vi "Configure Regions.vi"(8 "error in (no error)":errorcluster, 10 "regions":T1(array[cluster]), 11 "SOL Camera in":refnum<class "PL SOL Instruments Camera.lvclass">) -> (0 "error out":errorcluster, 3 "SOL Camera out":refnum<class "PL SOL Instruments Camera.lvclass">)   [LabVIEW 2015, in "PL SOL Instruments Camera.lvclass"]
doc: "Configures acquisition regions."
uses:
  PL SOL Instruments Camera.lvclass
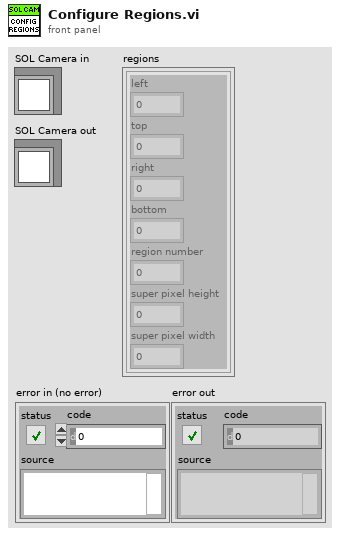
[diagram p1: front panel]
types:
  T1 = cluster{"left":u16, "top":u16, "right":u16, "bottom":u16, "region number":u16, "super pixel height":u16, "super pixel width":u16}[]
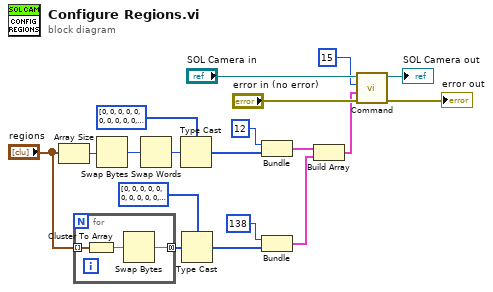
[diagram p0: block diagram]
diagram:
  n1 = Array Size(array="regions") -> (size(s)=w10:i32)
  n2 = for {
    tunnel: "regions" -> [w22] mode=indexing
    tunnel: [w20] -> w5 mode=concatenating
    n3 = Cluster To Array(cluster=w22) -> (array=w21:u16[])
    n4 = Swap Bytes(anything=w21) -> (byte swapped=w20:u16[])
  }
  n5 = Swap Bytes(anything=w10) -> (byte swapped=w12:i32)
  n6 = Swap Words(1:w12) -> (0:w11:i32)
  n7 = Type Cast(type=u8[] [0, 0, 0, 0, 0, 0, 0, 0, 0, 0, 0, 0, 0, 0, 0, 0, 0, 0, 0, 0, 0, 0, 0, 0, 0, 0, 0, 0, 0, 0, 0, 0, 0, 0, 0, 0, 0, 0, 0, 0, 0, 0, 0, 0, 0, 0, 0, 0, 0, 0, 0, 0, 0, 0, 0, 0, 0, 0, 0, 0, 0, 0, 0, 0, 0, 0, 0, 0, 0, 0, 0, 0, 0, 0, 0, 0, 0, 0, 0, 0, 0, 0, 0, 0, 0, 0, 0, 0, 0, 0, 0, 0, 0, 0, 0, 0, 0, 0, 0, 0, 4, 0, 0, 0, 0, 0, 0, 0, 0, 0, 0, 0, 0, 0, 0, 0, 0, 0, 0, 0, 0, 0, 0, 0, 0, 0, 0, 0, 0, 0, 0, 0, 0, 0, 0, 0, 0, 0, 0, 0, 0, 0, 0, 0, 0, 0, 0, 0, 0, 0, 0, 0, 0, 0, 0, 0, 0, 0, 0, 0, 0, 0, 0, 0, 0, 0, 0, 0, 0, 0, 0, 0, 0, 0, 0, 0, 0, 0, 0, 0, 0, 0, 0, 0, 0, 0, 0, 0, 0, 0, 0, 0, 0, 0, 0, 0, 0, 0, 0, 0, 0, 0, 0, 0, 0, 0, 0, 0, 0, 0, 0, 0, 0, 0, 0, 0, 0, 0, 0, 0, 0, 0, 0, 0] ("response"), x=w11) -> (*(type *) &x=w7:u8[])
  n8 = Type Cast(type=u8[] [0, 0, 0, 0, 0, 0, 0, 0, 0, 0, 0, 0, 0, 0, 0, 0, 0, 0, 0, 0, 0, 0, 0, 0, 0, 0, 0, 0, 0, 0, 0, 0, 0, 0, 0, 0, 0, 0, 0, 0, 0, 0, 0, 0, 0, 0, 0, 0, 0, 0, 0, 0, 0, 0, 0, 0, 0, 0, 0, 0, 0, 0, 0, 0, 0, 0, 0, 0, 0, 0, 0, 0, 0, 0, 0, 0, 0, 0, 0, 0, 0, 0, 0, 0, 0, 0, 0, 0, 0, 0, 0, 0, 0, 0, 0, 0, 0, 0, 0, 0, 4, 0, 0, 0, 0, 0, 0, 0, 0, 0, 0, 0, 0, 0, 0, 0, 0, 0, 0, 0, 0, 0, 0, 0, 0, 0, 0, 0, 0, 0, 0, 0, 0, 0, 0, 0, 0, 0, 0, 0, 0, 0, 0, 0, 0, 0, 0, 0, 0, 0, 0, 0, 0, 0, 0, 0, 0, 0, 0, 0, 0, 0, 0, 0, 0, 0, 0, 0, 0, 0, 0, 0, 0, 0, 0, 0, 0, 0, 0, 0, 0, 0, 0, 0, 0, 0, 0, 0, 0, 0, 0, 0, 0, 0, 0, 0, 0, 0, 0, 0, 0, 0, 0, 0, 0, 0, 0, 0, 0, 0, 0, 0, 0, 0, 0, 0, 0, 0, 0, 0, 0, 0, 0, 0] ("response"), x=w5) -> (*(type *) &x=w4:u8[])
  n9 = Bundle("offset"=12, "response"=w7) -> (w8:cluster{"offset":i32, "response":u8[]})  [unwired: 1 in]
  n10 = Bundle("offset"=138, "response"=w4) -> (w14:cluster{"offset":i32, "response":u8[]})  [unwired: 1 in]
  n11 = Build Array(w8, w14) -> (w1:cluster{"offset":i32, "response":u8[]}[])
  n12 = call "Command.vi"("error in (no error)"="error in (no error)", "data"=w1, "command"=u8 15, "SOL Camera in"="SOL Camera in") -> ("error out"=→"error out":errorcluster, "SOL Camera out"=→"SOL Camera out":refnum<class "PL SOL Instruments Camera.lvclass">)  [unwired: 5 in, 1 out]
